vi "Calculate Perpendicular Line.vi"(10 "Angle (deg)":sgl, 11 "Perpendicular Line":T1) -> (3 "Cluster":cluster{cluster{sgl, sgl}, cluster{sgl, sgl}})   [LabVIEW 2019]
uses:
  <vilib>/vision/NI_Vision_Development_Module.lvlib
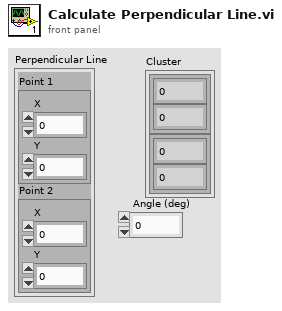
[diagram p1: front panel]
types:
  T1 = cluster{"Point 1":cluster{"X":sgl, "Y":sgl}, "Point 2":cluster{"X":sgl, "Y":sgl}}
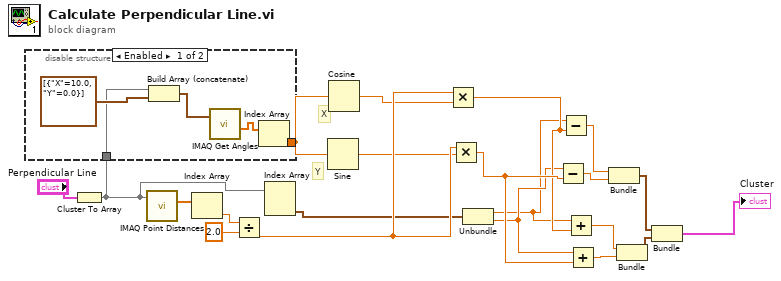
[diagram p0: block diagram]
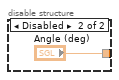
[diagram p2: hidden frame]
diagram:
  # "Y"
  # "X"
  n1 = Cluster To Array(cluster="Perpendicular Line") -> (array=w9:cluster{"X":sgl, "Y":sgl}[])
  n2 = disable-structure shown="Enabled" {
    disable-tunnel: [w26 "Angle (deg)"] -> w10
    disable-tunnel: w9 -> [w22 _]
    frame Enabled {
      n3 = Build Array (concatenate)(w22, cluster{"X":sgl, "Y":sgl}[] [{"X"=10.0, "Y"=0.0}] ("element")) -> (w24:cluster{"X":sgl, "Y":sgl}[])
      n4 = call "IMAQ Get Angles"("Points"=w24) -> ("Angles (rad)"=w25:sgl[])  [unwired: 4 in, 2 out]
      n5 = Index Array(array=w25) -> (element=w26:sgl)  [unwired: 1 in]
    }
    frame Disabled {
    }
  }
  n6 = call "IMAQ Point Distances"("Points"=w9) -> ("Distances"=w2:sgl[])  [unwired: 4 in, 1 out]
  n7 = Index Array(array=w2) -> (element=w6:sgl)  [unwired: 1 in]
  n8 = Divide(x=w6, y=sgl 2.0) -> (x/y=w11:sgl)
  n9 = Index Array(array=w9) -> (element #2=w5:cluster{"X":sgl, "Y":sgl})  [unwired: 2 in, 1 out]
  n10 = Sine(x=w10) -> (sin(x)=w8:sgl)
  n11 = Cosine(x=w10) -> (cos(x)=w7:sgl)
  n12 = Multiply(x=w11, y=w7) -> (x*y=w15:sgl)
  n13 = Multiply(x=w11, y=w8) -> (x*y=w16:sgl)
  n14 = Unbundle(w5) -> ("X"=w13:sgl, "Y"=w14:sgl)
  n15 = Subtract(x=w14, y=w16) -> (x-y=w4:sgl)
  n16 = Subtract(x=w13, y=w15) -> (x-y=w3:sgl)
  n17 = Add(x=w13, y=w15) -> (x+y=w18:sgl)
  n18 = Add(x=w14, y=w16) -> (x+y=w17:sgl)
  n19 = Bundle(w3, w4) -> (w19:cluster{sgl, sgl})  [unwired: 1 in]
  n20 = Bundle(w18, w17) -> (w20:cluster{sgl, sgl})  [unwired: 1 in]
  n21 = Bundle(w19, w20) -> (→"Cluster":cluster{cluster{sgl, sgl}, cluster{sgl, sgl}})  [unwired: 1 in]
